vi "FindNameInColorsArray(SubVI).vi"(1 "Name in":string, 2 "Array":string[](array[string])) -> (0 "Does the array contain this name?":bool)   [LabVIEW 2018]
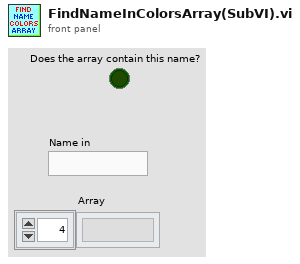
[diagram p1: front panel]
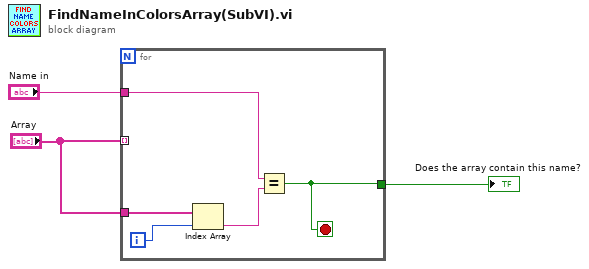
[diagram p0: block diagram]
diagram:
  n1 = for {
    tunnel: "Array" -> [_] mode=indexing
    tunnel: "Array" -> [w6]
    tunnel: "Name in" -> [w8]
    tunnel: [w7] -> w3
    i -> [w5]
    stop <- w7 stop-if-true
    n2 = Index Array(array=w6, index=w5) -> (element=w4:string)
    n3 = Equal?(x=w8, y=w4) -> (x = y?=w7:bool)
  }
  "Does the array contain this name?" <- w3
